vi "Rampa_Pos.vi"(0 "task/channels in":refnum<k21>, 1 "Start_A":dbl caption="Ángulo inicial" min=-5.0 max=5.0 step=0.05, 2 "Stop_A":dbl caption="Ángulo final" min=-5.0 max=5.0 step=0.05, 3 "Step_A":dbl=0.01 caption="Paso ángulo" min=0.01 max=1.0 step=0.05, 4 "ms to wait":u32=20 min=7 max=1000 step=1, 5 "Error In":errorcluster, 6 "# Ciclos":u16=1 min=1 max=20000 step=1) -> (19 "Error Out":errorcluster)   [LabVIEW 2016]
uses:
  Controles/Estados_RampaNEG.ctl
  <vilib>/DAQmx/write.llb/DAQmx Write (Analog DBL 1Chan 1Samp).vi
  <vilib>/DAQmx/miscellaneous.llb/DAQmx Fill In Error Info.vi
panel:
  out "OK":bool
  out "Volt":dbl caption="Voltaje (v)"
  in  "Cancel":bool
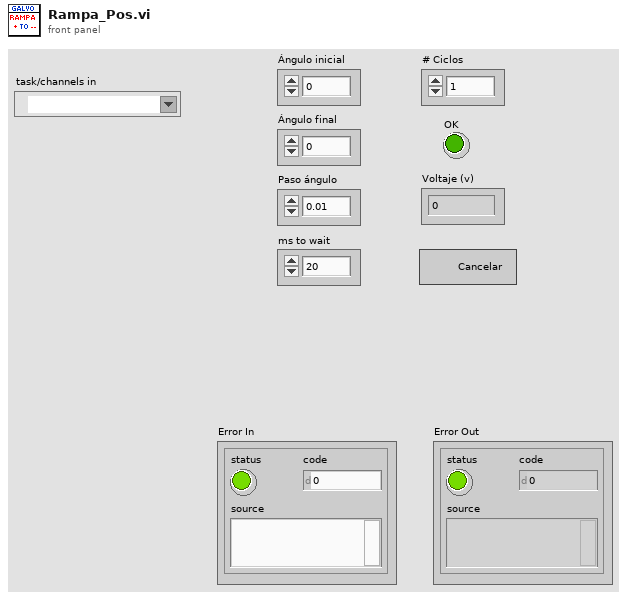
[diagram p1: front panel]
types:
  T1 = typedef "Estados_RampaNEG.ctl" = enum16{"Inicio", "Step+", "Ciclo+", "Step-", "Ciclo-"}
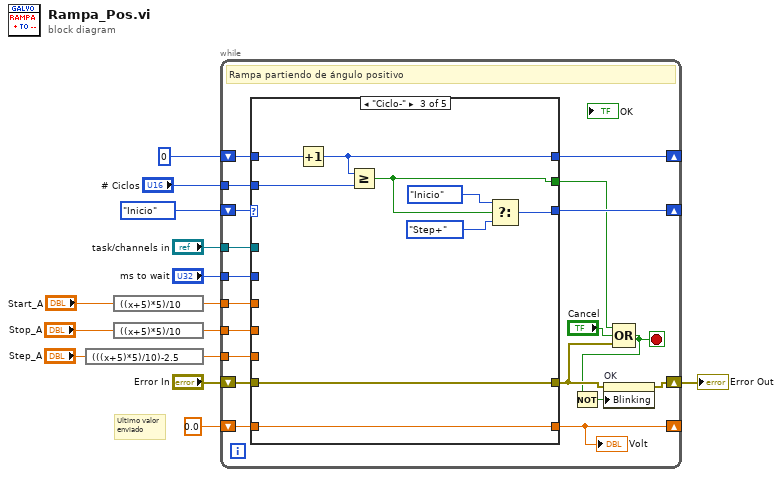
[diagram p0: block diagram]
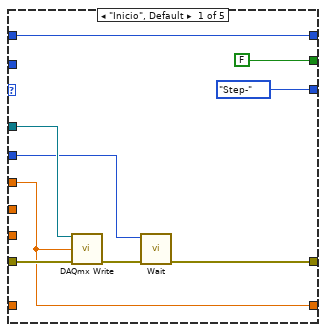
[diagram p2: hidden frame]
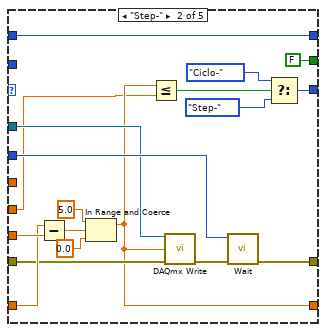
[diagram p3: hidden frame]
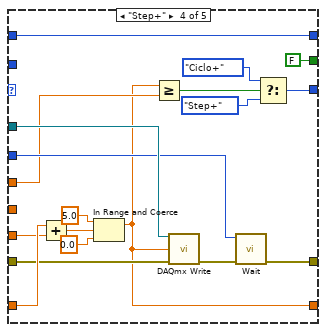
[diagram p4: hidden frame]
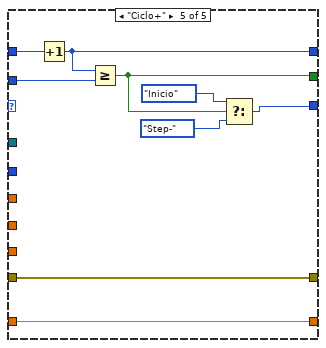
[diagram p5: hidden frame]
diagram:
  # "Ultimo valor\nenviado"
  n1 = expression code="(((x+5)*5)/10)-2.5"("Step_A") -> (w9:dbl)
  n2 = expression code="((x+5)*5)/10"("Start_A") -> (w11:dbl)
  n3 = expression code="((x+5)*5)/10"("Stop_A") -> (w10:dbl)
  n4 = while {
    tunnel: w11 -> [w32]
    tunnel: w10 -> [w31]
    tunnel: w9 -> [w30]
    shift-right: [w26] -> _
    shift-left: Estados_RampaNEG."Inicio" -> [w33]
    shift-right: [w21] -> w3
    shift-left: "Error In" -> [w29]
    tunnel: "task/channels in" -> [w28]
    tunnel: "ms to wait" -> [w27]
    shift-right: [w23] -> _
    shift-left: 0.0 ("Start_A") -> [w25]
    tunnel: "# Ciclos" -> [w18]
    shift-right: [w16] -> _
    shift-left: u16 0 -> [w17]
    stop <- w19 stop-if-true
    # "Rampa partiendo de ángulo positivo"
    n5 = case shown="\"Ciclo-\"" w33 {
      tunnel: w32 -> [w36 _ _ w73 _]
      tunnel: w31 -> [_ w45 _ _ _]
      tunnel: w30 -> [_ w60 _ w75 _]
      tunnel: w29 -> [w42 w58 w63 w86 w89]
      tunnel: w28 -> [w41 w50 _ w85 _]
      tunnel: [w38 w51 w63 w78 w89] -> w20
      tunnel: w27 -> [w39 w56 _ w83 _]
      tunnel: [Estados_RampaNEG."Step-" w55 w65 w82 w91] -> w26
      tunnel: [w36 w46 w64 w72 w88] -> w23
      tunnel: w25 -> [_ w59 w64 w87 w88]
      tunnel: w18 -> [_ _ w68 _ w95]
      tunnel: w17 -> [w35 w44 w69 w71 w96]
      tunnel: [w35 w44 w61 w71 w94] -> w16
      tunnel: [FALSE FALSE w62 FALSE w90] -> w15
      frame "Inicio", Default {
        n6 = call-poly <vilib>:"DAQmx Write.vi"("task/channels in"=w41, "data"=w36, "error in"=w42) -> ("error out"=w40:errorcluster)  [unwired: 10 in, 2 out]
        n7 = call "Wait.vi"("Error In"=w40, "ms to wait"=w39) -> ("Error Out"=w38:errorcluster)  [unwired: 9 in]
      }
      frame "Step-" {
        n8 = Subtract(x=w59, y=w60) -> (x-y=w47:dbl)
        n9 = In Range and Coerce(upper limit=5.0, x=w47, lower limit=0.0) -> (coerced(x)=w46:dbl)  [unwired: 1 out]
        n10 = Less Or Equal?(x=w46, y=w45) -> (x <= y?=w52:bool)
        n11 = call-poly <vilib>:"DAQmx Write.vi"("task/channels in"=w50, "data"=w46, "error in"=w58) -> ("error out"=w57:errorcluster)  [unwired: 10 in, 2 out]
        n12 = call "Wait.vi"("Error In"=w57, "ms to wait"=w56) -> ("Error Out"=w51:errorcluster)  [unwired: 9 in]
        n13 = Select(t=Estados_RampaNEG."Ciclo-", s=w52, f=Estados_RampaNEG."Step-") -> (s? t:f=w55:T1)
      }
      frame "Ciclo-" {
        n14 = Increment(x=w69) -> (x+1=w61:u16)
        n15 = Greater Or Equal?(x=w61, y=w68) -> (x >= y?=w62:bool)
        n16 = Select(t=Estados_RampaNEG."Inicio", s=w62, f=Estados_RampaNEG."Step+") -> (s? t:f=w65:T1)
      }
      frame "Step+" {
        n17 = Add(x=w87, y=w75) -> (x+y=w76:dbl)
        n18 = In Range and Coerce(upper limit=5.0, x=w76, lower limit=0.0) -> (coerced(x)=w72:dbl)  [unwired: 1 out]
        n19 = Greater Or Equal?(x=w72, y=w73) -> (x >= y?=w79:bool)
        n20 = call-poly <vilib>:"DAQmx Write.vi"("task/channels in"=w85, "data"=w72, "error in"=w86) -> ("error out"=w84:errorcluster)  [unwired: 10 in, 2 out]
        n21 = call "Wait.vi"("Error In"=w84, "ms to wait"=w83) -> ("Error Out"=w78:errorcluster)  [unwired: 9 in]
        n22 = Select(t=Estados_RampaNEG."Ciclo+", s=w79, f=Estados_RampaNEG."Step+") -> (s? t:f=w82:T1)
      }
      frame "Ciclo+" {
        n23 = Increment(x=w96) -> (x+1=w94:u16)
        n24 = Greater Or Equal?(x=w94, y=w95) -> (x >= y?=w90:bool)
        n25 = Select(t=Estados_RampaNEG."Inicio", s=w90, f=Estados_RampaNEG."Step-") -> (s? t:f=w91:T1)
      }
    }
    "Volt" <- w23
    n26 = Compound Arithmetic op=OR(w15, "Cancel", w20) -> (w19:bool)
    n27 = Not(x=w19) -> (.not. x?=w22:bool)
    n28 = property on="OK" class="Bool (strict)"(error in=w20, "Blinking"=w22) -> (error out=w21:errorcluster)  [unwired: 1 in, 1 out]
  }
  "Error Out" <- w3
